vi "MPC.vi"() -> ()   [LabVIEW 2021]
doc: "This example illustrates the use of MPC inside a Simulation Loop. This example does not include a state estimator. All states are measured directly from the plant. The entire setpoint profile is provided at one time to the Simulation Loop."
uses:
  <vilib>/addons/Control Design/_MPC/NI_CD_MPC.lvlib
  <vilib>/Simulation/Implementation/XNodeFramework/SimXNode/SimX.xnode
  <vilib>/addons/Control Design/_Utility/NI_CD_Model Viewer.lvlib
  <vilib>/addons/Control Design/_Model Construction/Model Typedefs.llb/CD General Elements.ctl
  <vilib>/addons/Control Design/_Model Construction/NI_LinSys_Model Typedefs.lvlib
  <vilib>/addons/Control Design/_Model Construction/Model Typedefs.llb/CD State Space Model (MIMO).ctl
  <vilib>/Simulation/DiscreteLinear/Implementation/NILVSim Discrete State Space Direct.llb/SIM Discrete State Space Direct Diagram (CD).vi
  <vilib>/addons/Control Design/_Utility/Model Viewer.llb/Model Viewer SubVI/cd_Draw State-Space Equation (SS).vi
  <vilib>/addons/Control Design/_MPC/Build Controller/CD Create MPC Controller (Barrier).vi
  <vilib>/addons/Control Design/_MPC/Implement Controller/CD Implement MPC Controller (MIMO).vi
  <vilib>/addons/Control Design/_MPC/Datatypes/CD Cost Weight Parameters.ctl
  <vilib>/addons/Control Design/_MPC/Datatypes/CD Controller Parameters.ctl
panel:
  out "MV":dbl(graph)=1.8819455250701138e-06
  in  "Stop":bool
  out "PV":cluster{"Numeric":dbl, "setpoint":dbl}(graph)={"Numeric"=3.872843199958187e-06, "setpoint"=0.0}
  in  "Tab Control":T1(tab)
  in  "State-Space Model":T2={"properties"={"Model name"="", "Input names"=[], "Output names"=[], "Input Delays"=[], "Output Delays"=[], "Sampling Time"=500.0, "Notes"=""}, "A"=[[-0.2]], "B"=[[2.0]], "C"=[[1.0]], "D"=[[0.0]], "StateNames"=[], "Transport Delay"=[]} {"Transport Delay" format="%.2f"; "D" format="%#.2g"; "C" format="%#.2g"; "B" format="%#.2g"; "A" format="%#.2g"; "properties"."Sampling Time" format="%#.6p"; "properties"."Output Delays" format="%.4f"; "properties"."Input Delays" format="%.4f"}
  out "x(k+1)":dbl[](array[numeric])=[2.98932241014859e-06] format="%.2f"
  in  "Ts [s]":dbl=0.1
  in  "Set-Point Profile":cluster{"time (s)":dbl, "Reference":dbl}[](array[cluster])=[{"time (s)"=0.0, "Reference"=0.0}, {"time (s)"=5.0, "Reference"=1.0}, {"time (s)"=15.0, "Reference"=0.0}] {"Reference" format="%.2f"; "time (s)" format="%.3f"}
  in  "MPC Controller Parameters":T4={"Initial Window"=0, "Prediction Horizon"=10, "Control Horizon"=10, "Integral Action?"=TRUE}
  in  "Final Time (s)":dbl=100.0
  in  "MPC Constraints (Barrier)":T5={"u min init"=[0.0], "u max final"=[5.0], "u min final"=[0.0], "u max init"=[5.0], "y max final"=[], "y min init"=[], "y min final"=[], "y max init"=[], "du max final"=[], "du min init"=[], "du min final"=[], "du max init"=[], "u min tolerance"=[], "u min penalty"=[], "u max tolerance"=[], "u max penalty"=[], "y min tolerance"=[], "y min penalty"=[], "y max tolerance"=[], "y max penalty"=[], "du min tolerance"=[], "du min penalty"=[], "du max tolerance"=[], "du max penalty"=[]} {"du max penalty" format="%.2f"; "du max tolerance" format="%.1e"; "du min penalty" format="%.2f"; "du min tolerance" format="%.1e"; "y max penalty" format="%.2f"; "y max tolerance" format="%.1e"; "y min penalty" format="%.2f"; "y min tolerance" format="%.1e"; "u max penalty" format="%.2f"; "u max tolerance" format="%.1e"; "u min penalty" format="%.2f"; "u min tolerance" format="%.1e"; "du max init" format="%.2f"; "du min final" format="%.2f"; "du min init" format="%.2f"; "du max final" format="%.2f"; "y max init" format="%.2f"; "y min final" format="%.2f"; "y min init" format="%.2f"; "y max final" format="%.2f"; "u max init" format="%.2f"; "u min final" format="%.2f"; "u min init" format="%.2f"; "u max final" format="%.2f"}
  in  "MPC Cost Weights":T6={"Output Error Weightings"=[[1.0]], "Control Action Change Weightings"=[[40.0]], "Control Action Error Weightings"=[], "Output Error Factors"=[], "Control Action Change Factors"=[], "Control Action Error Factors"=[]} {"Control Action Error Factors" format="%.2f"; "Control Action Change Factors" format="%.2f"; "Output Error Factors" format="%.2f"; "Control Action Error Weightings" format="%.2f"; "Control Action Change Weightings" format="%.2f"; "Output Error Weightings" format="%.2f"}
  in  "Error in (no error)":errorcluster
  out "Error out":errorcluster
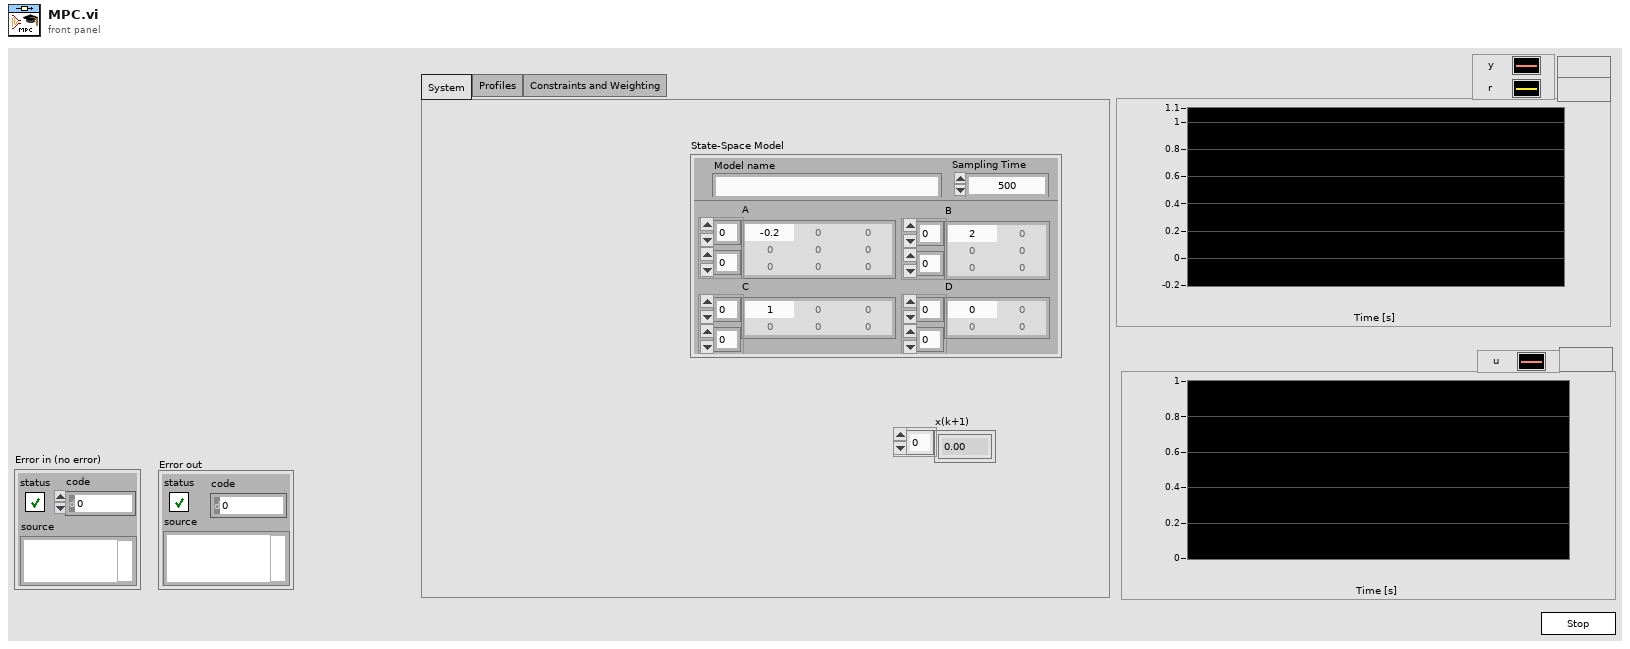
[diagram p1: front panel]
types:
  T1 = enum32{"System", "Profiles", "Constraints and Weighting"}
  T2 = typedef "NI_LinSys_Model Typedefs.lvlib/CD State Space Model (MIMO).ctl" = cluster{"properties":T3, "A":dbl[][], "B":dbl[][], "C":dbl[][], "D":dbl[][], "StateNames":string[], "Transport Delay":dbl[][]}
  T3 = typedef "NI_LinSys_Model Typedefs.lvlib/CD General Elements.ctl" = cluster{"Model name":string, "Input names":string[], "Output names":string[], "Input Delays":dbl[], "Output Delays":dbl[], "Sampling Time":dbl, "Notes":string}
  T4 = typedef "NI_CD_MPC.lvlib/CD Controller Parameters.ctl" = cluster{"Initial Window":i32, "Prediction Horizon":i32, "Control Horizon":i32, "Integral Action?":bool}
  T5 = cluster{"u min init":dbl[], "u max final":dbl[], "u min final":dbl[], "u max init":dbl[], "y max final":dbl[], "y min init":dbl[], "y min final":dbl[], "y max init":dbl[], "du max final":dbl[], "du min init":dbl[], "du min final":dbl[], "du max init":dbl[], "u min tolerance":dbl[], "u min penalty":dbl[], "u max tolerance":dbl[], "u max penalty":dbl[], "y min tolerance":dbl[], "y min penalty":dbl[], "y max tolerance":dbl[], "y max penalty":dbl[], "du min tolerance":dbl[], "du min penalty":dbl[], "du max tolerance":dbl[], "du max penalty":dbl[]}
  T6 = typedef "NI_CD_MPC.lvlib/CD Cost Weight Parameters.ctl" = cluster{"Output Error Weightings":dbl[][], "Control Action Change Weightings":dbl[][], "Control Action Error Weightings":dbl[][], "Output Error Factors":dbl[], "Control Action Change Factors":dbl[], "Control Action Error Factors":dbl[]}
  T7 = typedef "NI_CD_MPC.lvlib/CD MPC Model.ctl" = cluster{"H ":dbl[][], "G":dbl[][], "#Inputs":i32, "#Outputs":i32, "#States":i32, "#Disturbances":i32, "Integral Action?":bool, "Initial Data":T8, "Control Horizon":i32, "Prediction Horizon":i32, "Stopping Criteria":T9, "Inequality Constraints":T10, "Constraints":u16, "Initial Window":i32, "Internal Estimator?":bool, "L":dbl[][], "Plant Model (SS)":T2, "parameter bounds":cluster{"Xmin":dbl[], "Xmax":dbl[]}, "Sample Time":dbl, "Augmented SS Model":T2, "D":dbl[][], "K":dbl[][], "LN_y":dbl[][], "Inequality Constraints Barrier":T11, "H ^-1":dbl[][]}
  T8 = typedef "NI_CD_MPC.lvlib/CD MPC Data.ctl" = cluster{"Control Action (u)":dbl[], "Output (y)":dbl[], "Disturbance (d)":dbl[], "State (x)":dbl[], "Control Action Change (Du)":dbl[]}
  T9 = typedef "NI_Gmath.lvlib/stopping criteria.ctl" = cluster{"function tolerance":dbl, "parameter tolerance":dbl, "max iterations":i32, "max function calls":i32, "gradient tolerance":dbl, "max time (sec)":dbl}
  T10 = typedef "NI_CD_MPC.lvlib/CD Inequality Constraints and Parameter Bounds.ctl" = cluster{"Y max":dbl[], "Y min":dbl[], "U max":dbl[], "U min":dbl[], "tolerance":dbl}
  T11 = typedef "NI_CD_MPC.lvlib/CD Inequality Constraints and Parameter Bounds Barrier.ctl" = cluster{"Y max":dbl[], "Y min":dbl[], "U max":dbl[], "U min":dbl[], "dU max":dbl[], "dU min":dbl[], "pen min":dbl[], "tol min":dbl[], "pen max":dbl[], "tol max":dbl[]}
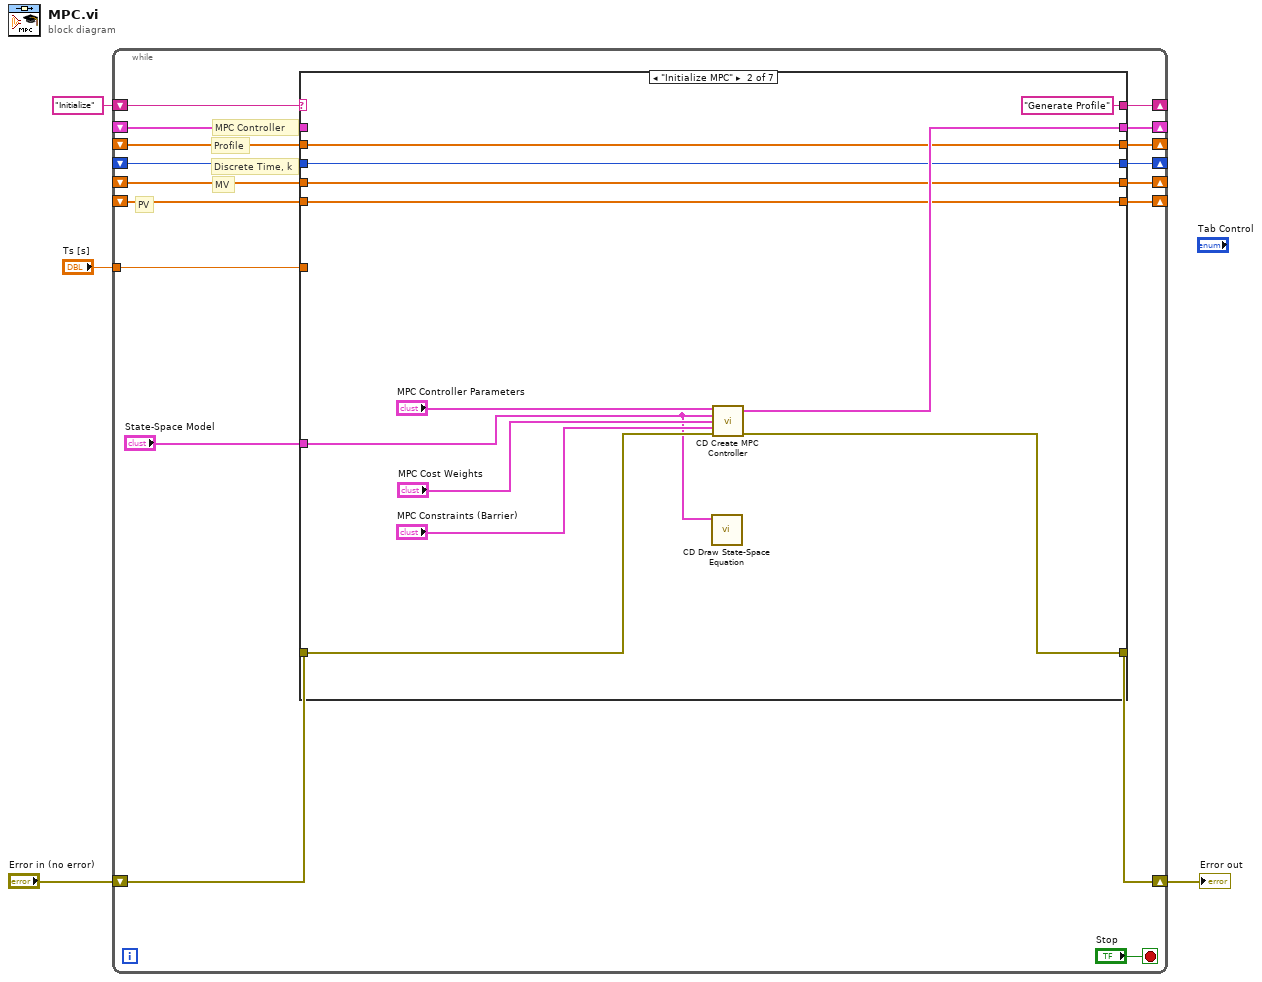
[diagram p0: block diagram]
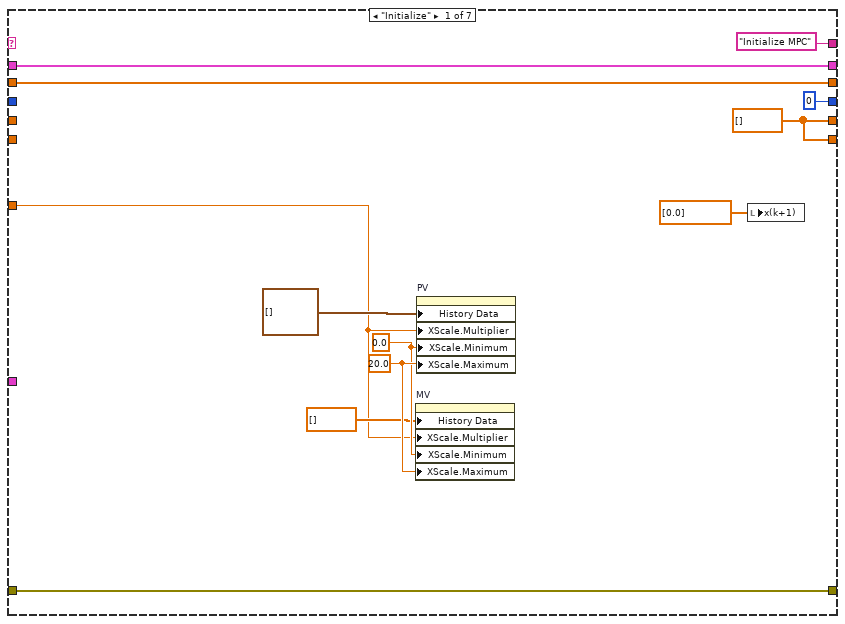
[diagram p2: hidden frame]
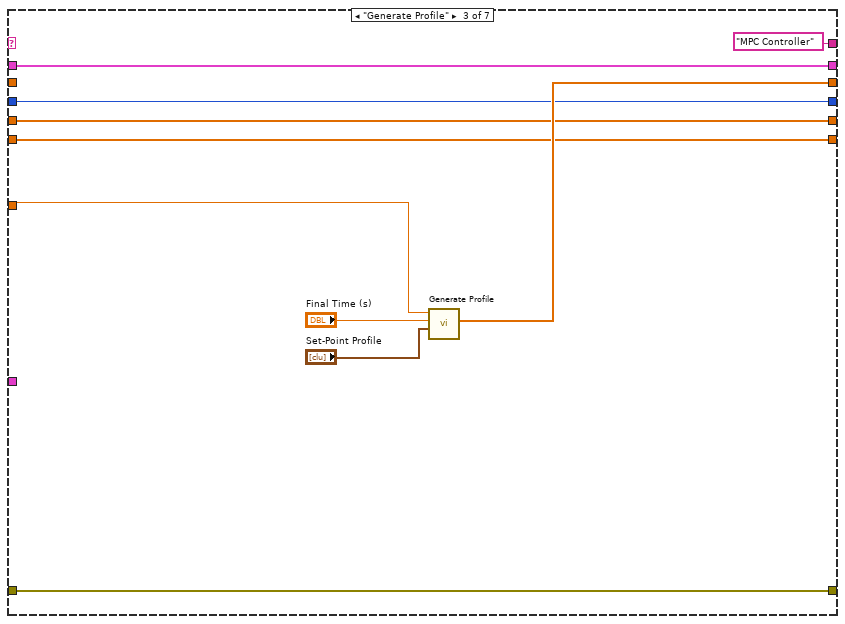
[diagram p3: hidden frame]
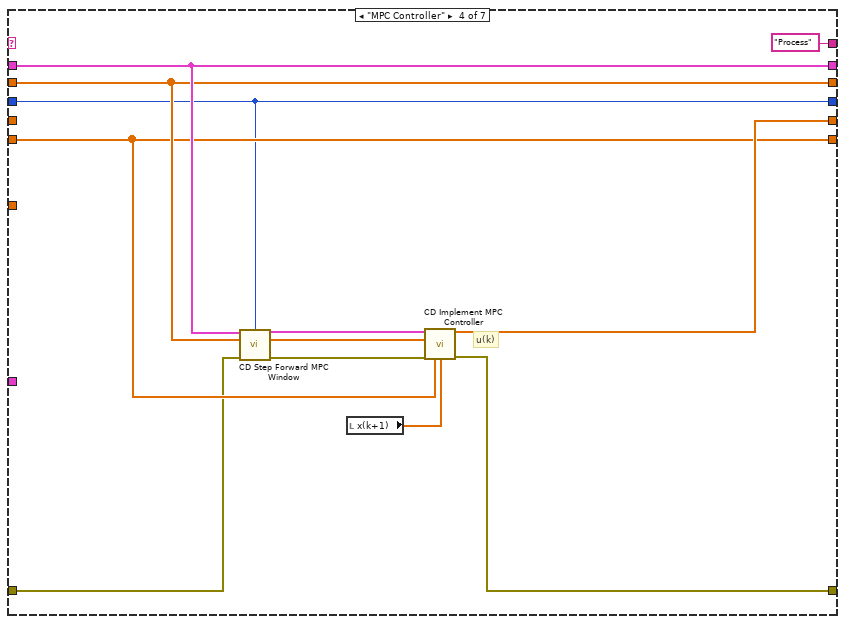
[diagram p4: hidden frame]
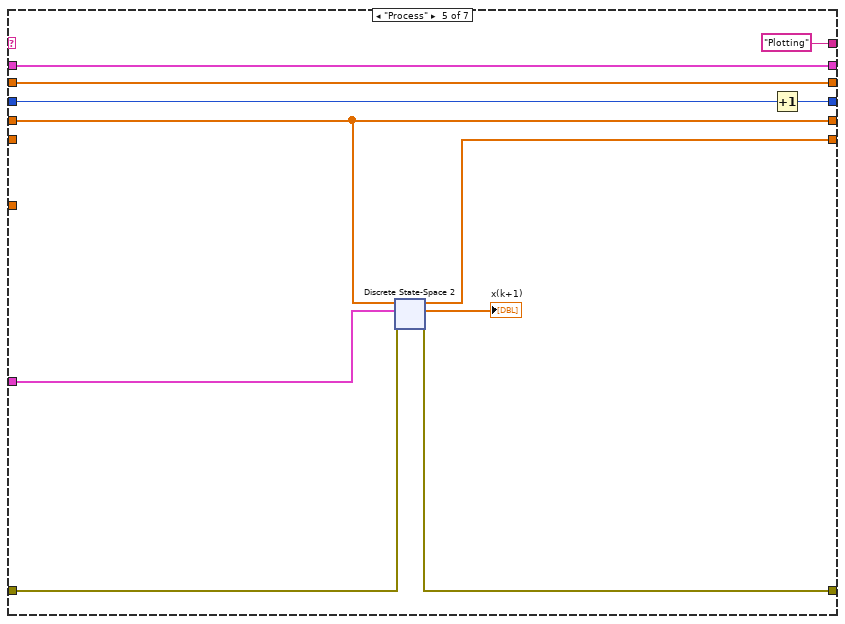
[diagram p5: hidden frame]
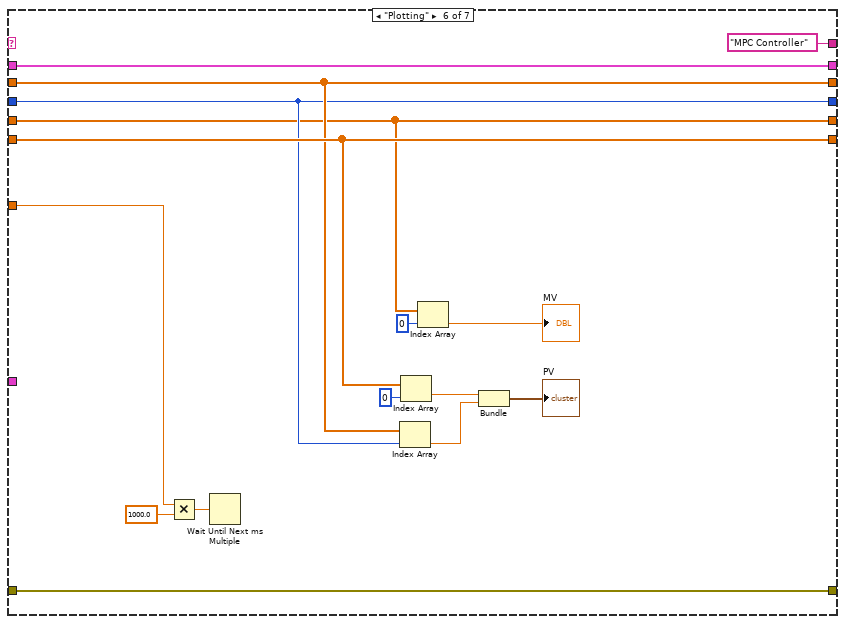
[diagram p6: hidden frame]
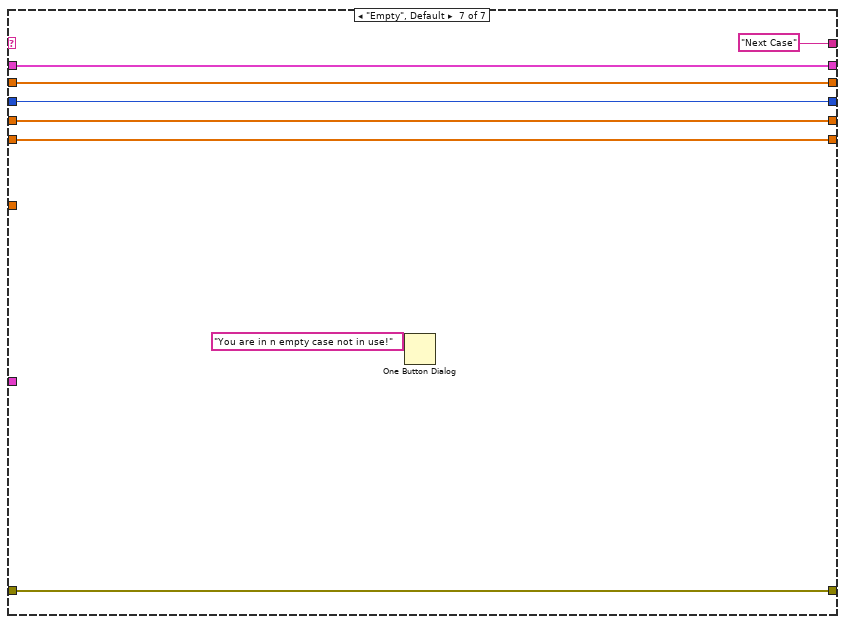
[diagram p7: hidden frame]
diagram:
  n1 = while {
    shift-right: [w18] -> _
    shift-left: "Initialize" -> [w21]
    tunnel: "Ts [s]" -> [w19]
    shift-right: [w16] -> w1
    shift-left: "Error in (no error)" -> [w17]
    shift-right: [w14] -> _
    shift-left: _ -> [w15]
    shift-right: [w13] -> _
    shift-left: _ -> [w12]
    shift-right: [w11] -> _
    shift-left: _ -> [w10]
    shift-right: [w9] -> _
    shift-left: _ -> [w8]
    shift-right: [w7] -> _
    shift-left: _ -> [w6]
    stop <- "Stop" stop-if-true
    # "PV"
    # "MV"
    # "Discrete Time, k"
    # "Profile"
    # "MPC Controller"
    n2 = case shown="\"Initialize MPC\"" w21 {
      tunnel: w19 -> [w29 _ w47 _ _ w91 _]
      tunnel: ["Initialize MPC" "Generate Profile" "MPC Controller" "Process" "Plotting" "MPC Controller" "Next Case"] -> w18
      tunnel: w17 -> [w27 w42 w56 w59 w74 w103 w111]
      tunnel: [w27 w41 w56 w58 w73 w103 w111] -> w16
      tunnel: w15 -> [w26 _ w55 w64 w79 w102 w110]
      tunnel: [w26 w40 w55 w64 w79 w102 w110] -> w14
      tunnel: [w25 w38 w51 w63 w77 w94 w108] -> w13
      tunnel: w12 -> [w25 w38 _ w63 w77 w94 w108]
      tunnel: [0 w37 w50 w57 w69 w93 w107] -> w11
      tunnel: w10 -> [_ w37 w50 w57 w70 w93 w107]
      tunnel: [w23 w36 w49 w62 w76 w89 w106] -> w9
      tunnel: w8 -> [_ w36 w49 _ w76 w89 w106]
      tunnel: [w23 w35 w48 w61 w72 w96 w105] -> w7
      tunnel: w6 -> [_ w35 w48 w61 _ w96 w105]
      tunnel: "State-Space Model" -> [_ w34 _ _ w75 _ _]
      frame "Initialize" {
        w23 = dbl[] []
        w33 = 20.0 ("X Scale.Range:Maximum")
        w32 = 0.0 ("X Scale.Range:Minimum")
        n3 = property on="MV" class="WFChart (strict)"("History Data"=dbl[] [], "XScale.Multiplier"=w29, "XScale.Minimum"=w32, "XScale.Maximum"=w33) -> ()  [unwired: 2 in, 2 out]
        n4 = property on="PV" class="WFChart (strict)"("History Data"=cluster{"Numeric":dbl, "setpoint":dbl}[] [], "XScale.Multiplier"=w29, "XScale.Minimum"=w32, "XScale.Maximum"=w33) -> ()  [unwired: 2 in, 2 out]
        n5 = local write "x(k+1)"(dbl[] [0.0] ("x(k+1)")) -> ()
      }
      frame "Initialize MPC" {
        n6 = call-poly <vilib>:"CD Draw State-Space Equation.vi"("State-Space Model"=w34) -> ("Equation"=w44:picture)  [unwired: 8 in, 2 out]
        n7 = call-poly <vilib>:"CD Create MPC Controller.vi"("MPC Controller Parameters"="MPC Controller Parameters", "State-Space Model"=w34, "MPC Cost Weights"="MPC Cost Weights", "MPC Constraints (Barrier)"="MPC Constraints (Barrier)", "error in (no error)"=w42) -> ("MPC Controller"=w40:T7, "error out"=w41:errorcluster)  [unwired: 9 in]
      }
      frame "Generate Profile" {
        n8 = call "Generate Profile.vi"("Set-Point Profile"="Set-Point Profile", "Final Time (s)"="Final Time (s)", "Ts (s)"=w47) -> ("Profile"=w51:dbl[])  [unwired: 8 in]
      }
      frame "MPC Controller" {
        # "u(k)"
        n9 = call <vilib>:"CD Step Forward MPC Window.vi"("MPC Controller In"=w64, "Timestep Index"=w57, "Interleaved Output Setpoint"=w63, "error in (no error)"=w59) -> ("MPC Controller Out"=w65:T7, "Output Reference Window"=w66:dbl[], "error out"=w67:errorcluster)  [unwired: 6 in, 3 out]
        n10 = local read "x(k+1)"() -> (w60:dbl[])
        n11 = call-poly <vilib>:"CD Implement MPC Controller.vi"("MPC Controller"=w65, "Output Reference Window"=w66, "error in (no error)"=w67, "Measured Output y(k)"=w61, "Estimated State xhat(k)"=w60) -> ("Control Action u(k)"=w62:dbl[], "error out"=w58:errorcluster)  [unwired: 6 in, 3 out]
      }
      frame "Process" {
        n12 = xnode ("Discrete State-Space 2")("input u(k)"=w76, "State-Space"=w75, "error in (no error)"=w74) -> ("state x(k+1)"=→"x(k+1)":dbl[], "output y(k)"=w72:dbl[], "error out"=w73:errorcluster)  [unwired: 1 in, 1 out]
        n13 = Increment(x=w70) -> (x+1=w69:i32)
      }
      frame "Plotting" {
        n14 = Multiply(x=w91, y=1000.0) -> (x*y=w98:dbl)
        n15 = Wait Until Next ms Multiple(millisecond multiple=w98) -> ()  [unwired: 1 out]
        n16 = Index Array(array=w94, index=w93) -> (element=w92:dbl)
        n17 = Index Array(array=w96, index=0) -> (element=w95:dbl)
        n18 = Index Array(array=w89, index=0) -> (element=→"MV":dbl)
        n19 = Bundle("Numeric"=w95, "Numeric"=w92) -> (→"PV":cluster{"Numeric":dbl, "Numeric":dbl})  [unwired: 1 in]
      }
      frame "Empty", Default {
        n20 = One Button Dialog(message="You are in n empty case not in use!") -> ()  [unwired: 1 in, 1 out]
      }
    }
  }
  "Error out" <- w1
